vi "Forward Tell.vi"(8 "Error in":errorcluster, 10 "Msg DVR":refnum<data-value>, 11 "TEMPLATE Actor in":refnum<class "TEMPLATE Actor.lvclass">) -> (0 "Error out":errorcluster, 3 "TEMPLATE Actor out":refnum<class "TEMPLATE Actor.lvclass">)   [LabVIEW 2020, in "_Template.lvlib" / "Templates.lvlib" / "TEMPLATE jettl Actor.lvlib" / "TEMPLATE Actor.lvlib" / "TEMPLATE Actor.lvclass"]
uses:
  jettl/jettl/Msg/Msg.lvclass
  jettl/jettl/Msg Contents/Msg Contents.lvclass
  TEMPLATE Actor.lvclass
  TEMPLATE Actor.lvclass/TEMPLATE Actor.ctl
  jettl/jettl/Unified Actor Relation.ctl
  jettl/jettl/jettl.lvlib
  jettl/jettl/Teller.ctl
  jettl/jettl/Msg.ctl
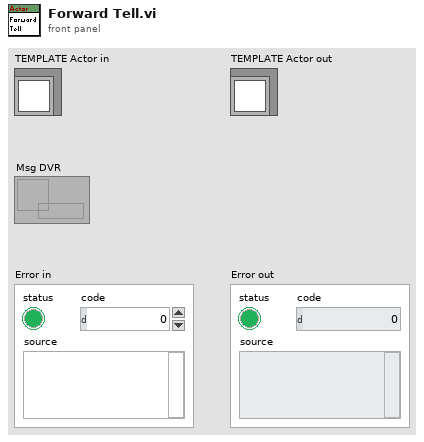
[diagram p1: front panel]
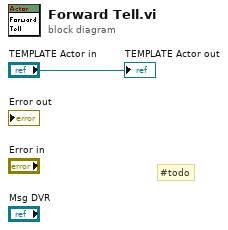
[diagram p0: block diagram]
diagram:
  # "#todo"
  "TEMPLATE Actor out" <- "TEMPLATE Actor in"
